vi "Test ArduinoMicro.vi"(5 "Enable":bool=TRUE, 8 "error in":errorcluster, 11 "VISA resource name":refnum<visa-resource-name>="COM25") -> (0 "error out":errorcluster)   [LabVIEW 2013]
uses:
  Controles/P2018 Arduino Control.ctl
  ArduinoMicro Module Control.ctl
  P2022 TB INCAR GLOBALES.vi
panel:
  out "Status":bool
  out "write string":string
  in  "ESTADO":T1
  out "read string":string
  out "Timeout":bool
  in  "stop":bool
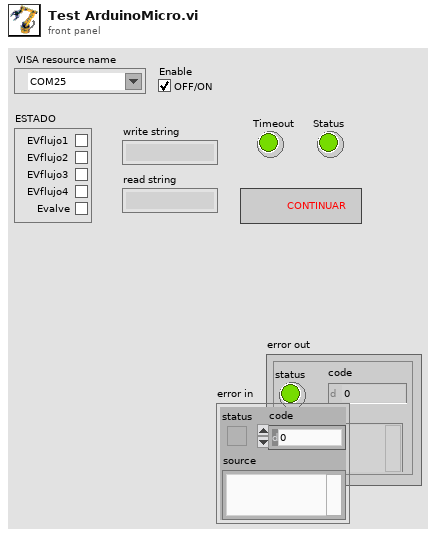
[diagram p1: front panel]
types:
  T1 = typedef "P2018 Arduino Control.ctl" = cluster{"EVflujo1":bool, "EVflujo2":bool, "EVflujo3":bool, "EVflujo4":bool, "Evalve":bool}
  T2 = typedef "ArduinoMicro Module Control.ctl" = enum16{"Initialize", "Read Data", "Write Data", "Enable", "Disable", "Shutdown"}
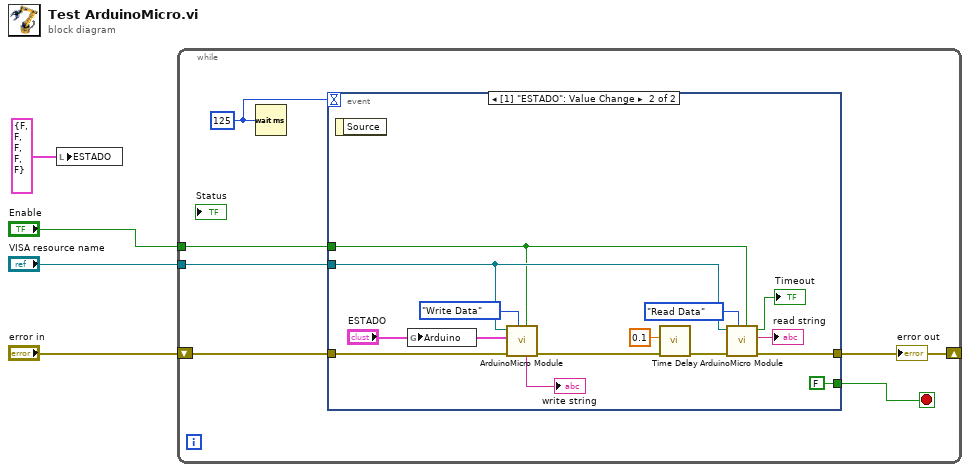
[diagram p0: block diagram]
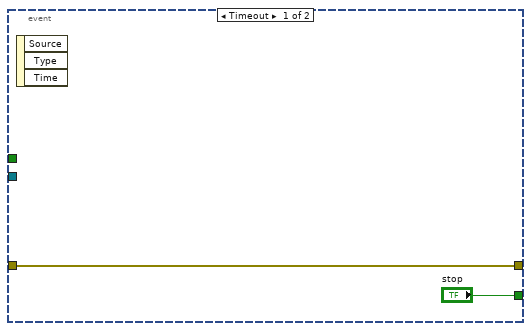
[diagram p2: hidden frame]
diagram:
  n1 = local write "ESTADO"(T1 {"EVflujo1"=FALSE, "EVflujo2"=FALSE, "EVflujo3"=FALSE, "EVflujo4"=FALSE, "Evalve"=FALSE} ("ESTADO")) -> ()
  n2 = while {
    shift-right: [w8] -> _
    shift-left: "error in" -> [w7]
    tunnel: "VISA resource name" -> [w9]
    tunnel: "Enable" -> [w10]
    stop <- w6 stop-if-true
    w5 = u32 125 ("milliseconds to wait")
    n3 = Wait (ms)(milliseconds to wait=w5) -> ()  [unwired: 1 out]
    n4 = event shown="[1] \"ESTADO\": Value Change" {
      selector: _ -> [_ _]
      dyn-events: _ -> [_ _]
      timeout: w5 -> [_ _]
      tunnel: w10 -> [_ w17]
      tunnel: w9 -> [_ w18]
      tunnel: [w12 w16] -> w8
      tunnel: w7 -> [w12 w15]
      tunnel: ["stop" FALSE ("stop")] -> w6
      event Timeout {
        n5 = event-data() -> ()  [unwired: 1 in, 3 out]
      }
      event Value Change {
        n6 = event-data() -> ()  [unwired: 1 in, 1 out]
        n7 = global write "P2022 TB INCAR GLOBALES.vi" "Arduino"("ESTADO") -> ()
        n8 = call "ArduinoMicro Module.vi"("Enable"=w17, "Command"=ArduinoMicro_Module_Control."Write Data", "error in (no error)"=w15, "VALVES"="ESTADO", "VISA resource name"=w18) -> ("error out"=w25:errorcluster, "write string"=→"write string":string)  [unwired: 2 in, 3 out]
        n9 = call "Time Delay"("error in (no error)"=w25, "Delay Time (s)"=0.1) -> ("error out"=w26:errorcluster)  [unwired: 9 in]
        n10 = call "ArduinoMicro Module.vi"("Enable"=w17, "Command"=ArduinoMicro_Module_Control."Read Data", "error in (no error)"=w26, "VISA resource name"=w18) -> ("error out"=w16:errorcluster, "read string"=→"read string":string, "TimeOut"=→"Timeout":bool)  [unwired: 3 in, 2 out]
      }
    }
    "error out" <- w8
  }
